vi "Coord window-Normalise coord for display.vi"(10 "MCList ItemNames":string[][](array[string]), 11 "Bounds":T1) -> (3 "Normalised coordinates (for display)":cluster{"x":i16, "y":i16}[](array[cluster]))   [LabVIEW 2020]
uses:
  <vilib>/Utility/miscctls.llb/LVBoundsTypeDef.ctl
  Globals/Coord window-Globals.vi
  <vilib>/gmath/NI_Gmath.lvlib
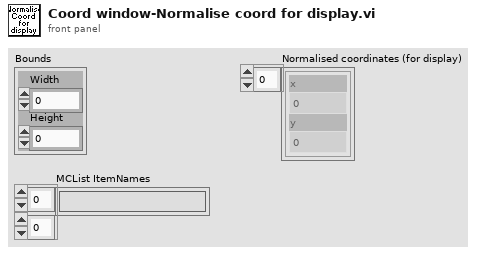
[diagram p1: front panel]
types:
  T1 = typedef "LVBoundsTypeDef.ctl" = cluster{"Width":u32, "Height":u32}
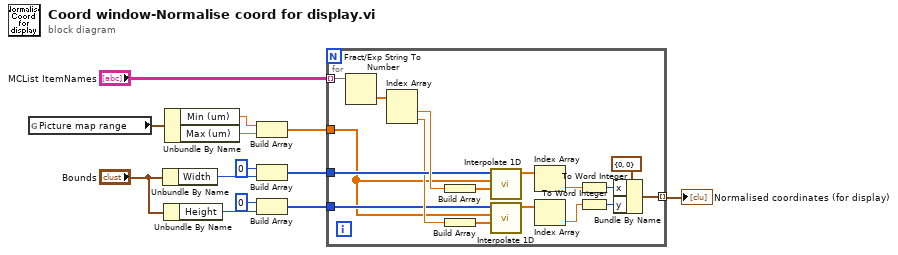
[diagram p0: block diagram]
diagram:
  n1 = global read "Coord window-Globals.vi" "Picture map range"() -> (w4:cluster{"Min (um)":dbl, "Max (um)":dbl})
  n2 = Unbundle By Name("Bounds") -> ("Width"=w5:u32)
  n3 = Unbundle By Name("Bounds") -> ("Height"=w8:u32)
  n4 = Unbundle By Name(w4) -> ("Min (um)"=w3:dbl, "Max (um)"=w2:dbl)
  n5 = Build Array(w3, w2) -> (w1:dbl[])
  n6 = Build Array(u32 0 ("element"), w5) -> (w9:u32[])
  n7 = Build Array(u32 0 ("element"), w8) -> (w10:u32[])
  n8 = for {
    tunnel: "MCList ItemNames" -> [w30] mode=indexing
    tunnel: w9 -> [w22]
    tunnel: w1 -> [w16]
    tunnel: [w23] -> w11 mode=indexing
    tunnel: w10 -> [w17]
    n9 = Fract/Exp String To Number(string=w30) -> (number=w29:dbl[])  [unwired: 3 in, 1 out]
    n10 = Index Array(array=w29) -> (element #1=w27:dbl, element #2=w19:dbl)  [unwired: 2 in]
    n11 = Build Array(w27) -> (w28:dbl[])
    n12 = Build Array(w19) -> (w20:dbl[])
    n13 = call <vilib>:"Interpolate 1D.vi"("xi"=w28, "X"=w16, "Y"=w22) -> ("yi"=w26:dbl[])  [unwired: 6 in, 2 out]
    n14 = call <vilib>:"Interpolate 1D.vi"("xi"=w20, "X"=w16, "Y"=w17) -> ("yi"=w21:dbl[])  [unwired: 6 in, 2 out]
    n15 = Index Array(array=w26) -> (element=w24:dbl)  [unwired: 1 in]
    n16 = Index Array(array=w21) -> (element=w18:dbl)  [unwired: 1 in]
    n17 = To Word Integer(number=w24) -> (16bit integer=w15:i16)
    n18 = To Word Integer(number=w18) -> (16bit integer=w14:i16)
    n19 = Bundle By Name(cluster=cluster{"x":i16, "y":i16} {"x"=0, "y"=0} ("point(x,y)"), "x"=w15, "y"=w14) -> (w23:cluster{"x":i16, "y":i16})
  }
  "Normalised coordinates (for display)" <- w11
